vi "Upload a file.vi"() -> ()   [LabVIEW 2011]
doc: "This example shows you how you can upload a file from your local filesystem to one of your Amazon S3 buckets."
uses:
  Typedefs/Access_Key_Type.ctl
  Typedefs/Secret_Key_Type.ctl
  vi.lib/National Instruments/LabVIEW Interface for Amazon S3/Typedefs/AMZ_S3_AWS Credentials.ctl
  vi.lib/National Instruments/LabVIEW Interface for Amazon S3/Typedefs/AMZ_S3_ACL.ctl
  vi.lib/National Instruments/LabVIEW Interface for Amazon S3/Typedefs/AMZ_S3_API_PUT Object Request Parameters.ctl
  vi.lib/National Instruments/LabVIEW Interface for Amazon S3/Typedefs/AMZ_S3_Storage Class.ctl
  vi.lib/National Instruments/LabVIEW Interface for Amazon S3/Typedefs/AMZ_S3_Object Metadata.ctl
  vi.lib/National Instruments/LabVIEW Interface for Amazon S3/Typedefs/AMZ_S3_API_POST Multipart Object Request Parameters.ctl
  vi.lib/National Instruments/LabVIEW Interface for Amazon S3/LV Interface for Amazon S3.lvlib
panel:
  in  "Secret Key":T1
  in  "Access Key":T2
  out "Location":string caption="New object's location"
  in  "Make public?":bool
  in  "Stop":bool
  in  "Upload":bool
  in  "Object Path":string
  out "Selected bucket":string
  # "To use this VI, you have to register first with Amazon to have an Amazon AWS account.\nIf you don't have an account yet, go to http://aws.amazon.com and Create an AWS account!"
  # "Note: You have to own at least one bucket to be able to use this VI!\n1. Fill in your AWS Credentials\n2. Run this VI\n3. Select the file you want to upload in the pop-up dialog\n4. Select one of your buckets you want to use in the pop-up dialog\n5. Modify the Object path if you want to upload to another location\n6. Set \"Make public?\" to the value you want\n7. Press the Upload button to start the upload process\n8. If the upload is successful, you will see the New object's location"
  # "Note: If you do not make an object public, you won't be able to download it using the\nlink provided in the New object's location indicator.\nThat's because you have to authenticate yourself to access non-public objects."
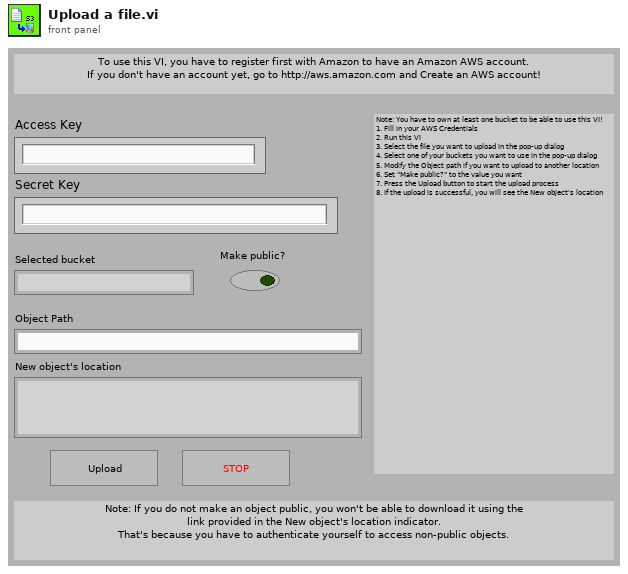
[diagram p1: front panel]
types:
  T1 = typedef "Secret_Key_Type.ctl" = string
  T2 = typedef "Access_Key_Type.ctl" = string
  T3 = typedef "LV Interface for Amazon S3.lvlib/AMZ_S3_AWS Credentials.ctl" = cluster{"Access Key":string, "Secret Key":string}
  T4 = typedef "LV Interface for Amazon S3.lvlib/AMZ_S3_ACL.ctl" = enum16{"private", "public-read", "public-read-write", "authenticated-read", "bucket-owner-read", "bucket-owner-full-control"}
  T5 = typedef "LV Interface for Amazon S3.lvlib/AMZ_S3_API_PUT Object Request Parameters.ctl" = cluster{"Content Type":string, "ACL":T4, "Storage Class":T6, "User Metadata":T7[], "Content MD5":string}
  T6 = typedef "LV Interface for Amazon S3.lvlib/AMZ_S3_Storage Class.ctl" = enum16{"STANDARD", "REDUCED_REDUNDANCY"}
  T7 = typedef "LV Interface for Amazon S3.lvlib/AMZ_S3_Object Metadata.ctl" = cluster{"Key":string, "Value":string}
  T8 = typedef "LV Interface for Amazon S3.lvlib/AMZ_S3_API_POST Multipart Object Request Parameters.ctl" = cluster{"Content Type":string, "ACL":T4, "Storage Class":T6, "User Metadata":T7[]}
  T9 = typedef "LV Interface for Amazon S3.lvlib/AMZ_S3_API_Bucket.ctl" = cluster{"Name":string, "CreationDate":timestamp}
  T10 = typedef "LV Interface for Amazon S3.lvlib/AMZ_S3_API_CompleteMultipartUploadResult.ctl" = cluster{"Location":string, "Bucket":string, "Key":string, "ETag":string}
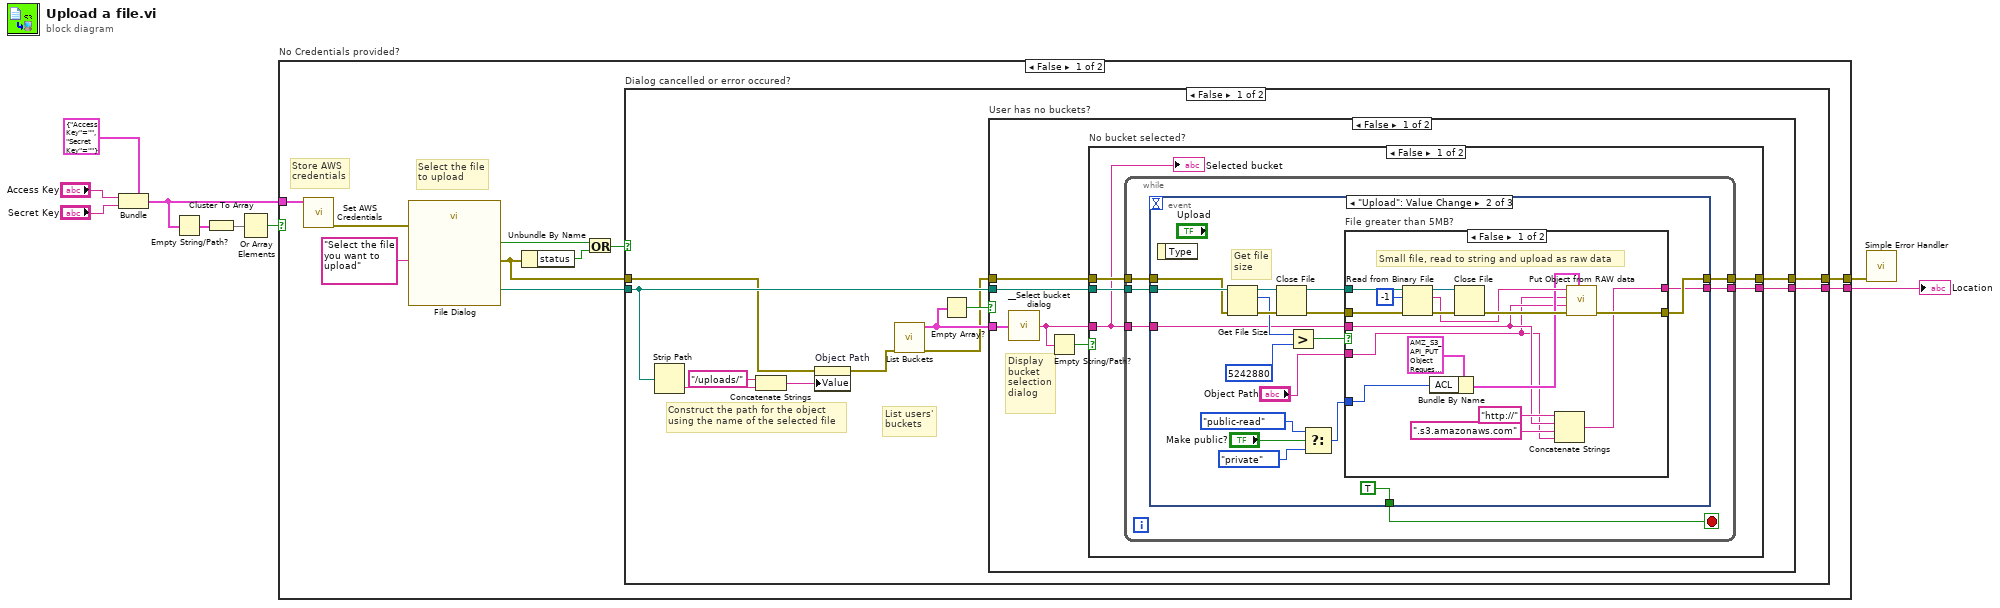
[diagram p0: block diagram]
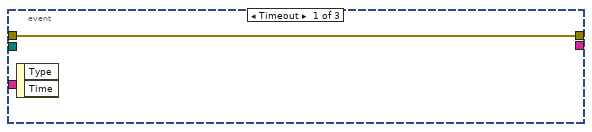
[diagram p2: hidden frame]
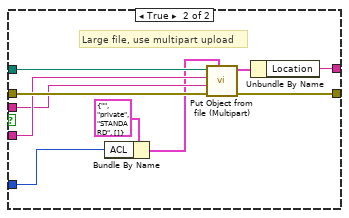
[diagram p3: hidden frame]
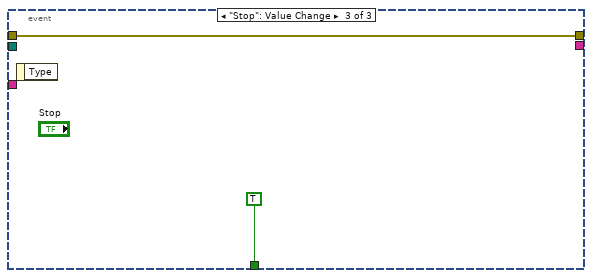
[diagram p4: hidden frame]
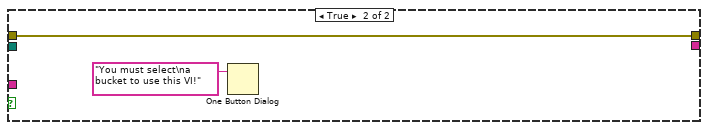
[diagram p5: hidden frame]
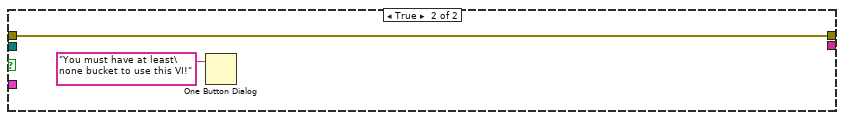
[diagram p6: hidden frame]
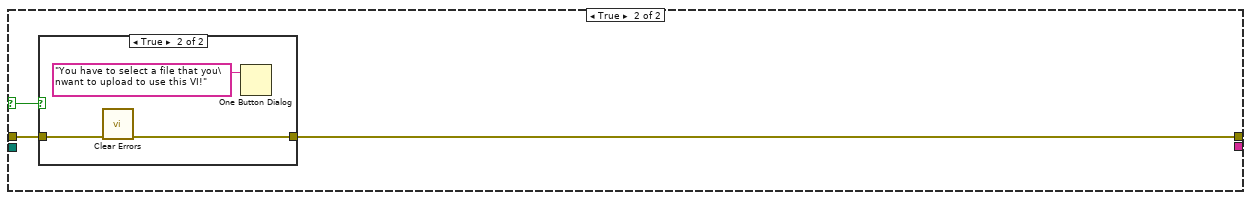
[diagram p7: hidden frame]
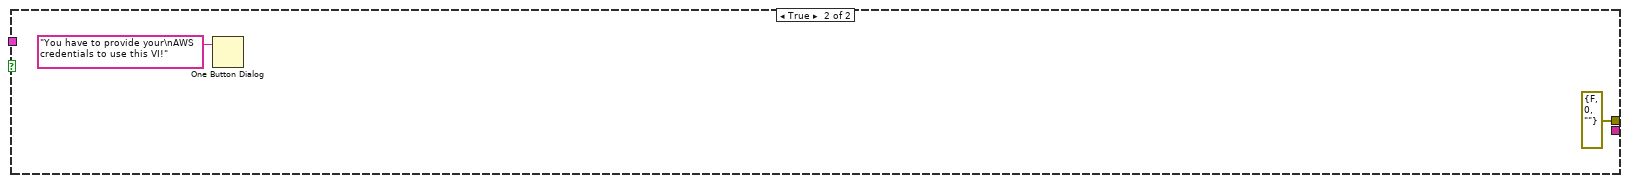
[diagram p9: hidden frame]
diagram:
  n1 = Bundle(cluster=T3 {"Access Key"="", "Secret Key"=""} ("AWS Credentials in"), "Access Key"="Access Key", "Secret Key"="Secret Key") -> (w1:T3)
  n2 = Empty String/Path?(string/path=w1) -> (empty?=w9:cluster{"Access Key":bool, "Secret Key":bool})
  n3 = Cluster To Array(cluster=w9) -> (array=w8:bool[])
  n4 = Or Array Elements(Boolean array=w8) -> (logical OR=w7:bool)
  n5 = case "No Credentials provided?" shown="False" w7 {
    tunnel: w1 -> [w19 _]
    tunnel: [w11 errorcluster {"status"=FALSE, "code"=0, "source"=""} ("error out")] -> w6
    tunnel: [w10 _] -> w5
    frame False {
      # "Select the file\nto upload"
      # "Store AWS\ncredentials"
      n6 = call "Set AWS Credentials.vi"("AWS Credentials in"=w19) -> ("error out"=w18:errorcluster)  [unwired: 10 in]
      n7 = call "File Dialog"("prompt"="Select the file you want to upload", "error in"=w18) -> ("selected path"=w12:path, "cancelled"=w15:bool, "error out"=w13:errorcluster)  [unwired: 10 in, 1 out]
      n8 = Unbundle By Name(w13) -> ("status"=w16:bool)
      n9 = Or(x=w15, y=w16) -> (x .or. y?=w14:bool)
      n10 = case "Dialog cancelled or error occured?" shown="False" w14 {
        selector: w14 -> [_ w102]
        tunnel: w13 -> [w23 w101]
        tunnel: w12 -> [w24 _]
        tunnel: [w22 w100] -> w11
        tunnel: [w20 _] -> w10
        frame False {
          # "List users'\nbuckets"
          # "Construct the path for the object\nusing the name of the selected file"
          n11 = Strip Path(path=w24) -> (name=w30:string)  [unwired: 1 out]
          n12 = Concatenate Strings("/uploads/" ("string"), w30) -> (w28:string)
          n13 = property on="Object Path" class="Str"(error in=w23, "Value"=w28) -> (error out=w27:errorcluster)  [unwired: 1 in, 1 out]
          n14 = call "List Buckets.vi"("error in (no error)"=w27) -> ("error out"=w21:errorcluster, "Buckets"=w25:T9[])  [unwired: 9 in]
          n15 = Empty Array?(array=w25) -> (empty?=w26:bool)
          n16 = case "User has no buckets?" shown="False" w26 {
            tunnel: w25 -> [w37 _]
            tunnel: w24 -> [w32 _]
            tunnel: w21 -> [w34 w98]
            tunnel: [w33 w98] -> w22
            tunnel: [w31 _] -> w20
            frame False {
              # "Display\nbucket\nselection\ndialog"
              n17 = call "__Select bucket dialog.vi"("Buckets"=w37) -> ("Selected bucket"=w35:string)
              n18 = Empty String/Path?(string/path=w35) -> (empty?=w36:bool)
              n19 = case "No bucket selected?" shown="False" w36 {
                tunnel: w35 -> [w38 _]
                tunnel: w34 -> [w41 w96]
                tunnel: [w40 w96] -> w33
                tunnel: w32 -> [w42 _]
                tunnel: [w39 _] -> w31
                frame False {
                  n20 = while {
                    tunnel: w42 -> [w47]
                    tunnel: w41 -> [w48]
                    tunnel: [w45] -> w40
                    tunnel: w38 -> [w44]
                    tunnel: [w43] -> w39
                    stop <- w46 stop-if-true
                    n21 = event shown="[1] \"Upload\": Value Change" {
                      selector: _ -> [_ _ _]
                      dyn-events: _ -> [_ _ _]
                      timeout: _ -> [_ _ _]
                      tunnel: w48 -> [w49 w65 w95]
                      tunnel: w47 -> [_ w66 _]
                      tunnel: [_ TRUE TRUE] -> w46
                      tunnel: [w49 w51 w95] -> w45
                      tunnel: w44 -> [_ w57 _]
                      tunnel: [_ w50 _] -> w43
                      event Timeout {
                        n22 = event-data() -> ()  [unwired: 1 in, 2 out]
                      }
                      event "Upload": Value Change {
                        # "Get file\nsize"
                        n23 = event-data() -> ()  [unwired: 1 in, 1 out]
                        n24 = Get File Size(file=w66, error in=w65) -> (refnum out=w63:refnum<file>, size (in bytes)=w62:i64, 0:w64:errorcluster)
                        n25 = Close File(refnum=w63, error in=w64) -> (path=w58:path, error out=w59:errorcluster)
                        n26 = Greater?(x=w62, y=i64 5242880) -> (0:w60:bool)
                        n27 = Select(t=AMZ_S3_ACL."public-read" ("ACL"), s="Make public?", f=AMZ_S3_ACL."private" ("ACL")) -> (s? t:f=w52:T4)
                        n28 = case "File greater than 5MB?" shown="False" w60 {
                          tunnel: w59 -> [w83 w93]
                          tunnel: w58 -> [w82 w92]
                          tunnel: w57 -> [w70 w90]
                          tunnel: "Object Path" -> [w69 w91]
                          tunnel: w52 -> [w75 w85]
                          tunnel: [w73 w89] -> w51
                          tunnel: [w68 w87] -> w50
                          frame False {
                            # "Small file, read to string and upload as raw data"
                            n29 = Read from Binary File(8:w83, 10:-1 ("count (1)"), 11:w82) -> (0:w80:errorcluster, 2:w77:string, 3:w79:refnum<file>)  [unwired: 3 in, 1 out]
                            n30 = Bundle By Name(cluster=T5 {"Content Type"="", "ACL"=enum."private", "Storage Class"=enum."STANDARD", "User Metadata"=[], "Content MD5"=""} ("Request Parameters"), "ACL"=w75) -> (w74:T5)
                            n31 = Close File(refnum=w79, error in=w80) -> (error out=w78:errorcluster)  [unwired: 1 out]
                            n32 = Concatenate Strings("http://" ("string"), w70, ".s3.amazonaws.com" ("string"), w69) -> (w68:string)
                            n33 = call "Put Object from RAW data.vi"("Request Parameters"=w74, "error in (no error)"=w78, "Bucket"=w70, "Path"=w69, "Data"=w77) -> ("error out"=w73:errorcluster)  [unwired: 5 in, 1 out]
                          }
                          frame True {
                            # "Large file, use multipart upload"
                            n34 = Bundle By Name(cluster=T8 {"Content Type"="", "ACL"=enum."private", "Storage Class"=enum."STANDARD", "User Metadata"=[]} ("Request Parameters"), "ACL"=w85) -> (w84:T8)
                            n35 = call "Put Object from file (Multipart).vi"("Request Parameters"=w84, "error in (no error)"=w93, "Bucket"=w90, "Object path"=w91, "Local file path"=w92) -> ("error out"=w89:errorcluster, "CompleteMultipartUploadResult"=w88:T10)  [unwired: 4 in, 1 out]
                            n36 = Unbundle By Name(w88) -> ("Location"=w87:string)
                          }
                        }
                      }
                      event "Stop": Value Change {
                        n37 = event-data() -> ()  [unwired: 1 in, 1 out]
                      }
                    }
                  }
                  "Selected bucket" <- w38
                }
                frame True {
                  n38 = One Button Dialog(message="You must select\na bucket to use this VI!") -> ()  [unwired: 1 in, 1 out]
                }
              }
            }
            frame True {
              n39 = One Button Dialog(message="You must have at least\none bucket to use this VI!") -> ()  [unwired: 1 in, 1 out]
            }
          }
        }
        frame True {
          n40 = case shown="True" w102 {
            tunnel: w101 -> [w103 w105]
            tunnel: [w103 w104] -> w100
            frame False {
            }
            frame True {
              n41 = call <vilib>:"Clear Errors.vi"("error in (no error)"=w105) -> ("error out"=w104:errorcluster)  [unwired: 6 in]
              n42 = One Button Dialog(message="You have to select a file that you\nwant to upload to use this VI!") -> ()  [unwired: 1 in, 1 out]
            }
          }
        }
      }
    }
    frame True {
      n43 = One Button Dialog(message="You have to provide your\nAWS credentials to use this VI!") -> ()  [unwired: 1 in, 1 out]
    }
  }
  "Location" <- w5
  n44 = call <vilib>:"Simple Error Handler.vi"("error in (no error)"=w6) -> ()  [unwired: 4 in, 5 out]
